vi "GeoData.vi"() -> ()   [LabVIEW 2017] (continued)
\t6079\tSan luis obispo\tCA\tSan Luis Obispo County\tH1\n93445\t6079\tOceano\tCA\tSan Luis Obispo County\tH1\n93421\t6079\tArroyo grande\tCA\tSan Luis Obispo County\tH1\n93426\t6079\tBradley\tCA\tSan Luis Obispo County\tH1\n93443\t6079\tMorro bay\tCA\tSan Luis Obispo County\tH1\n93435\t6079\tHarmony\tCA\tSan Luis Obispo County\tH1\n93453\t6079\tSanta margarita\tCA\tSan Luis Obispo County\tH1\n93409\t6079\tSan luis obispo\tCA\tSan Luis Obispo County\tH1\n93428\t6079\tCambria\tCA\tSan Luis Obispo County\tH1\n93452\t6079\tSan simeon\tCA\tSan Luis Obispo County\tH1\n93424\t6079\tAvila beach\tCA\tSan Luis Obispo County\tH1\n93446\t6079\tPaso robles\tCA\tSan Luis Obispo County\tH1\n93430\t6079\tCayucos\tCA\tSan Luis Obispo County\tH1\n93444\t6079\tNipomo\tCA\tSan Luis Obispo County\tH1\n93408\t6079\tSan luis obispo\tCA\tSan Luis Obispo County\tH1\n93407\t6079\tSan luis obispo\tCA\tSan Luis Obispo County\tH1\n93410\t6079\tSan luis obispo\tCA\tSan Luis Obispo County\tH1\n93423\t6079\tAtascadero\tCA\tSan Luis Obispo County\tH1\n93449\t6079\tPismo beach\tCA\tSan Luis Obispo County\tH1\n93465\t6079\tTempleton\tCA\tSan Luis Obispo County\tH1\n93461\t6079\tShandon\tCA\tSan Luis Obispo County\tH1\n93254\t6079\tNew cuyama\tCA\tSan Luis Obispo County\tH1\n93405\t6079\tSan luis obispo\tCA\tSan Luis Obispo County\tH1\n93402\t6079\tLos osos\tCA\tSan Luis Obispo County\tH1\n93442\t6079\tMorro bay\tCA\tSan Luis Obispo County\tH1\n93422\t6079\tAtascadero\tCA\tSan Luis Obispo County\tH1\n93432\t6079\tCreston\tCA\tSan Luis Obispo County\tH1\n93403\t6079\tSan luis obispo\tCA\tSan Luis Obispo County\tH1\n93412\t6079\tLos osos\tCA\tSan Luis Obispo County\tH1\n93433\t6079\tGrover beach\tCA\tSan Luis Obispo County\tH1\n93454\t6079\tSanta maria\tCA\tSan Luis Obispo County\tH1\n93458\t6079\tSanta maria\tCA\tSan Luis Obispo County\tH1\n93252\t6079\tMaricopa\tCA\tSan Luis Obispo County\tH1\n93451\t6079\tSan miguel\tCA\tSan Luis Obispo County\tH1\n93447\t6079\tPaso robles\tCA\tSan Luis Obispo County\tH1\n93448\t6079\tPismo beach\tCA\tSan Luis Obispo County\tH1\n93483\t6079\tGrover beach\tCA\tSan Luis Obispo County\tH1\n93401\t6079\tSan luis obispo\tCA\tSan Luis Obispo County\tH1\n93475\t6079\tOceano\tCA\tSan Luis Obispo County\tH1\n94404\t6081\tSan mateo\tCA\tSan Mateo County\tH1\n94128\t6081\tSan francisco\tCA\tSan Mateo County\tH1\n94011\t6081\tBurlingame\tCA\tSan Mateo County\tH1\n94017\t6081\tDaly city\tCA\tSan Mateo County\tH1\n94080\t6081\tSouth san francisco\tCA\tSan Mateo County\tH1\n94070\t6081\tSan carlos\tCA\tSan Mateo County\tH1\n94014\t6081\tDaly city\tCA\tSan Mateo County\tH1\n94025\t6081\tMenlo park\tCA\tSan Mateo County\tH1\n94030\t6081\tMillbrae\tCA\tSan Mateo County\tH1\n94044\t6081\tPacifica\tCA\tSan Mateo County\tH1\n94065\t6081\tRedwood city\tCA\tSan Mateo County\tH1\n94497\t6081\tSan mateo\tCA\tSan Mateo County\tH1\n94066\t6081\tSan bruno\tCA\tSan Mateo County\tH1\n94027\t6081\tAtherton\tCA\tSan Mateo County\tH1\n94021\t6081\tLoma mar\tCA\tSan Mateo County\tH1\n94401\t6081\tSan mateo\tCA\tSan Mateo County\tH1\n94002\t6081\tBelmont\tCA\tSan Mateo County\tH1\n94010\t6081\tBurlingame\tCA\tSan Mateo County\tH1\n94028\t6081\tPortola valley\tCA\tSan Mateo County\tH1\n94063\t6081\tRedwood city\tCA\tSan Mateo County\tH1\n94125\t6081\tSan francisco\tCA\tSan Mateo County\tH1\n94303\t6081\tPalo alto\tCA\tSan Mateo County\tH1\n94134\t6081\tSan francisco\tCA\tSan Mateo County\tH1\n94015\t6081\tDaly city\tCA\tSan Mateo County\tH1\n94018\t6081\tEl granada\tCA\tSan Mateo County\tH1\n94074\t6081\tSan gregorio\tCA\tSan Mateo County\tH1\n94026\t6081\tMenlo park\tCA\tSan Mateo County\tH1\n94112\t6081\tSan francisco\tCA\tSan Mateo County\tH1\n94403\t6081\tSan mateo\tCA\tSan Mateo County\tH1\n94019\t6081\tHalf moon bay\tCA\tSan Mateo County\tH1\n94038\t6081\tMoss beach\tCA\tSan Mateo County\tH1\n94402\t6081\tSan mateo\tCA\tSan Mateo County\tH1\n94005\t6081\tBrisbane\tCA\tSan Mateo County\tH1\n94064\t6081\tRedwood city\tCA\tSan Mateo County\tH1\n94020\t6081\tLa honda\tCA\tSan Mateo County\tH1\n94061\t6081\tRedwood city\tCA\tSan Mateo County\tH1\n94062\t6081\tRedwood city\tCA\tSan Mateo County\tH1\n94037\t6081\tMontara\tCA\tSan Mateo County\tH1\n94083\t6081\tSouth san francisco\tCA\tSan Mateo County\tH1\n94060\t6081\tPescadero\tCA\tSan Mateo County\tH1\n93105\t6083\tSanta barbara\tCA\tSanta Barbara County\tH1\n93116\t6083\tGoleta\tCA\tSanta Barbara County\tH1\n93437\t6083\tLompoc\tCA\tSanta Barbara County\tH1\n93102\t6083\tSanta barbara\tCA\tSanta Barbara County\tH1\n93120\t6083\tSanta barbara\tCA\tSanta Barbara County\tH1\n93440\t6083\tLos alamos\tCA\tSanta Barbara County\tH1\n93427\t6083\tBuellton\tCA\tSanta Barbara County\tH1\n93101\t6083\tSanta barbara\tCA\tSanta Barbara County\tH1\n93118\t6083\tGoleta\tCA\tSanta Barbara County\tH1\n93160\t6083\tSanta barbara\tCA\tSanta Barbara County\tH1\n93441\t6083\tLos olivos\tCA\tSanta Barbara County\tH1\n93436\t6083\tLompoc\tCA\tSanta Barbara County\tH1\n93109\t6083\tSanta barbara\tCA\tSanta Barbara County\tH1\n93111\t6083\tSanta barbara\tCA\tSanta Barbara County\tH1\n93106\t6083\tSanta barbara\tCA\tSanta Barbara County\tH1\n93254\t6083\tNew cuyama\tCA\tSanta Barbara County\tH1\n93429\t6083\tCasmalia\tCA\tSanta Barbara County\tH1\n93013\t6083\tCarpinteria\tCA\tSanta Barbara County\tH1\n93455\t6083\tSanta maria\tCA\tSanta Barbara County\tH1\n93190\t6083\tSanta barbara\tCA\tSanta Barbara County\tH1\n93110\t6083\tSanta barbara\tCA\tSanta Barbara County\tH1\n93108\t6083\tSanta barbara\tCA\tSanta Barbara County\tH1\n93457\t6083\tSanta maria\tCA\tSanta Barbara County\tH1\n93438\t6083\tLompoc\tCA\tSanta Barbara County\tH1\n93014\t6083\tCarpinteria\tCA\tSanta Barbara County\tH1\n93434\t6083\tGuadalupe\tCA\tSanta Barbara County\tH1\n93454\t6083\tSanta maria\tCA\tSanta Barbara County\tH1\n93463\t6083\tSolvang\tCA\tSanta Barbara County\tH1\n93458\t6083\tSanta maria\tCA\tSanta Barbara County\tH1\n93456\t6083\tSanta maria\tCA\tSanta Barbara County\tH1\n93252\t6083\tMaricopa\tCA\tSanta Barbara County\tH1\n93117\t6083\tGoleta\tCA\tSanta Barbara County\tH1\n93130\t6083\tSanta barbara\tCA\tSanta Barbara County\tH1\n93150\t6083\tSanta barbara\tCA\tSanta Barbara County\tH1\n93464\t6083\tSolvang\tCA\tSanta Barbara County\tH1\n93460\t6083\tSanta ynez\tCA\tSanta Barbara County\tH1\n93103\t6083\tSanta barbara\tCA\tSanta Barbara County\tH1\n93140\t6083\tSanta barbara\tCA\tSanta Barbara County\tH1\n93121\t6083\tSanta barbara\tCA\tSanta Barbara County\tH1\n93067\t6083\tSummerland\tCA\tSanta Barbara County\tH1\n93199\t6083\tGoleta\tCA\tSanta Barbara County\tH1\n94550\t6085\tLivermore\tCA\tSanta Clara County\tH1\n94040\t6085\tMountain view\tCA\tSanta Clara County\tH1\n95033\t6085\tLos gatos\tCA\tSanta Clara County\tH1\n95111\t6085\tSan jose\tCA\tSanta Clara County\tH1\n95113\t6085\tSan jose\tCA\tSanta Clara County\tH1\n95132\t6085\tSan jose\tCA\tSanta Clara County\tH1\n95122\t6085\tSan jose\tCA\tSanta Clara County\tH1\n95138\t6085\tSan jose\tCA\tSanta Clara County\tH1\n95150\t6085\tSan jose\tCA\tSanta Clara County\tH1\n95172\t6085\tSan jose\tCA\tSanta Clara County\tH1\n95071\t6085\tSaratoga\tCA\tSanta Clara County\tH1\n95164\t6085\tSan jose\tCA\tSanta Clara County\tH1\n95109\t6085\tSan jose\tCA\tSanta Clara County\tH1\n95141\t6085\tSan jose\tCA\tSanta Clara County\tH1\n94089\t6085\tSunnyvale\tCA\tSanta Clara County\tH1\n94301\t6085\tPalo alto\tCA\tSanta Clara County\tH1\n95030\t6085\tLos gatos\tCA\tSanta Clara County\tH1\n95119\t6085\tSan jose\tCA\tSanta Clara County\tH1\n95121\t6085\tSan jose\tCA\tSanta Clara County\tH1\n95156\t6085\tSan jose\tCA\tSanta Clara County\tH1\n95101\t6085\tSan jose\tCA\tSanta Clara County\tH1\n94306\t6085\tPalo alto\tCA\tSanta Clara County\tH1\n94024\t6085\tLos altos\tCA\tSanta Clara County\tH1\n95035\t6085\tMilpitas\tCA\tSanta Clara County\tH1\n95070\t6085\tSaratoga\tCA\tSanta Clara County\tH1\n95129\t6085\tSan jose\tCA\tSanta Clara County\tH1\n95130\t6085\tSan jose\tCA\tSanta Clara County\tH1\n95127\t6085\tSan jose\tCA\tSanta Clara County\tH1\n95123\t6085\tSan jose\tCA\tSanta Clara County\tH1\n95153\t6085\tSan jose\tCA\tSanta Clara County\tH1\n95002\t6085\tAlviso\tCA\tSanta Clara County\tH1\n95154\t6085\tSan jose\tCA\tSanta Clara County\tH1\n94085\t6085\tSunnyvale\tCA\tSanta Clara County\tH1\n94304\t6085\tPalo alto\tCA\tSanta Clara County\tH1\n94028\t6085\tPortola valley\tCA\tSanta Clara County\tH1\n95037\t6085\tMorgan hill\tCA\tSanta Clara County\tH1\n95050\t6085\tSanta clara\tCA\tSanta Clara County\tH1\n95076\t6085\tWatsonville\tCA\tSanta Clara County\tH1\n95120\t6085\tSan jose\tCA\tSanta Clara County\tH1\n95118\t6085\tSan jose\tCA\tSanta Clara County\tH1\n95131\t6085\tSan jose\tCA\tSanta Clara County\tH1\n95170\t6085\tSan jose\tCA\tSanta Clara County\tH1\n95134\t6085\tSan jose\tCA\tSanta Clara County\tH1\n95135\t6085\tSan jose\tCA\tSanta Clara County\tH1\n95021\t6085\tGilroy\tCA\tSanta Clara County\tH1\n95011\t6085\tCampbell\tCA\tSanta Clara County\tH1\n95158\t6085\tSan jose\tCA\tSanta Clara County\tH1\n95157\t6085\tSan jose\tCA\tSanta Clara County\tH1\n94035\t6085\tMountain view\tCA\tSanta Clara County\tH1\n95191\t6085\tSan jose\tCA\tSanta Clara County\tH1\n95013\t6085\tCoyote\tCA\tSanta Clara County\tH1\n94087\t6085\tSunnyvale\tCA\tSanta Clara County\tH1\n94303\t6085\tPalo alto\tCA\tSanta Clara County\tH1\n95051\t6085\tSanta clara\tCA\tSanta Clara County\tH1\n95032\t6085\tLos gatos\tCA\tSanta Clara County\tH1\n95056\t6085\tSanta clara\tCA\tSanta Clara County\tH1\n95110\t6085\tSan jose\tCA\tSanta Clara County\tH1\n95124\t6085\tSan jose\tCA\tSanta Clara County\tH1\n95125\t6085\tSan jose\tCA\tSanta Clara County\tH1\n95044\t6085\tRedwood estates\tCA\tSanta Clara County\tH1\n95151\t6085\tSan jose\tCA\tSanta Clara County\tH1\n95155\t6085\tSan jose\tCA\tSanta Clara County\tH1\n95015\t6085\tCupertino\tCA\tSanta Clara County\tH1\n95055\t6085\tSanta clara\tCA\tSanta Clara County\tH1\n95103\t6085\tSan jose\tCA\tSanta Clara County\tH1\n94086\t6085\tSunnyvale\tCA\tSanta Clara County\tH1\n95008\t6085\tCampbell\tCA\tSanta Clara County\tH1\n94043\t6085\tMountain view\tCA\tSanta Clara County\tH1\n95054\t6085\tSanta clara\tCA\tSanta Clara County\tH1\n95112\t6085\tSan jose\tCA\tSanta Clara County\tH1\n95117\t6085\tSan jose\tCA\tSanta Clara County\tH1\n95136\t6085\tSan jose\tCA\tSanta Clara County\tH1\n95026\t6085\tHoly city\tCA\tSanta Clara County\tH1\n95009\t6085\tCampbell\tCA\tSanta Clara County\tH1\n94088\t6085\tSunnyvale\tCA\tSanta Clara County\tH1\n95052\t6085\tSanta clara\tCA\tSanta Clara County\tH1\n94042\t6085\tMountain view\tCA\tSanta Clara County\tH1\n94039\t6085\tMountain view\tCA\tSanta Clara County\tH1\n95192\t6085\tSan jose\tCA\tSanta Clara County\tH1\n94023\t6085\tLos altos\tCA\tSanta Clara County\tH1\n95046\t6085\tSan martin\tCA\tSanta Clara County\tH1\n95023\t6085\tHollister\tCA\tSanta Clara County\tH1\n95116\t6085\tSan jose\tCA\tSanta Clara County\tH1\n95126\t6085\tSan jose\tCA\tSanta Clara County\tH1\n95159\t6085\tSan jose\tCA\tSanta Clara County\tH1\n95036\t6085\tMilpitas\tCA\tSanta Clara County\tH1\n94020\t6085\tLa honda\tCA\tSanta Clara County\tH1\n95161\t6085\tSan jose\tCA\tSanta Clara County\tH1\n95152\t6085\tSan jose\tCA\tSanta Clara County\tH1\n94302\t6085\tPalo alto\tCA\tSanta Clara County\tH1\n94305\t6085\tStanford\tCA\tSanta Clara County\tH1\n94022\t6085\tLos altos\tCA\tSanta Clara County\tH1\n94041\t6085\tMountain view\tCA\tSanta Clara County\tH1\n95020\t6085\tGilroy\tCA\tSanta Clara County\tH1\n95014\t6085\tCupertino\tCA\tSanta Clara County\tH1\n95038\t6085\tMorgan hill\tCA\tSanta Clara County\tH1\n95128\t6085\tSan jose\tCA\tSanta Clara County\tH1\n95133\t6085\tSan jose\tCA\tSanta Clara County\tH1\n95148\t6085\tSan jose\tCA\tSanta Clara County\tH1\n95140\t6085\tMount hamilton\tCA\tSanta Clara County\tH1\n95031\t6085\tLos gatos\tCA\tSanta Clara County\tH1\n95173\t6085\tSan jose\tCA\tSanta Clara County\tH1\n95139\t6085\tSan jose\tCA\tSanta Clara County\tH1\n95108\t6085\tSan jose\tCA\tSanta Clara County\tH1\n95160\t6085\tSan jose\tCA\tSanta Clara County\tH1\n95106\t6085\tSan jose\tCA\tSanta Clara County\tH1\n95033\t6087\tLos gatos\tCA\tSanta Cruz County\tH1\n95010\t6087\tCapitola\tCA\tSanta Cruz County\tH1\n95061\t6087\tSanta cruz\tCA\tSanta Cruz County\tH1\n95017\t6087\tDavenport\tCA\tSanta Cruz County\tH1\n95077\t6087\tWatsonville\tCA\tSanta Cruz County\tH1\n95006\t6087\tBoulder creek\tCA\tSanta Cruz County\tH1\n95062\t6087\tSanta cruz\tCA\tSanta Cruz County\tH1\n95076\t6087\tWatsonville\tCA\tSanta Cruz County\tH1\n95019\t6087\tFreedom\tCA\tSanta Cruz County\tH1\n95007\t6087\tBrookdale\tCA\tSanta Cruz County\tH1\n95073\t6087\tSoquel\tCA\tSanta Cruz County\tH1\n95041\t6087\tMount hermon\tCA\tSanta Cruz County\tH1\n95060\t6087\tSanta cruz\tCA\tSanta Cruz County\tH1\n95065\t6087\tSanta cruz\tCA\tSanta Cruz County\tH1\n95003\t6087\tAptos\tCA\tSanta Cruz County\tH1\n95005\t6087\tBen lomond\tCA\tSanta Cruz County\tH1\n95018\t6087\tFelton\tCA\tSanta Cruz County\tH1\n95001\t6087\tAptos\tCA\tSanta Cruz County\tH1\n95067\t6087\tScotts valley\tCA\tSanta Cruz County\tH1\n95066\t6087\tScotts valley\tCA\tSanta Cruz County\tH1\n95063\t6087\tSanta cruz\tCA\tSanta Cruz County\tH1\n94060\t6087\tPescadero\tCA\tSanta Cruz County\tH1\n95064\t6087\tSanta cruz\tCA\tSanta Cruz County\tH1\n96001\t6089\tRedding\tCA\tShasta County\tH1\n96022\t6089\tCottonwood\tCA\tShasta County\tH1\n96062\t6089\tMillville\tCA\tShasta County\tH1\n96076\t6089\tPlatina\tCA\tShasta County\tH1\n96099\t6089\tRedding\tCA\tShasta County\tH1\n96051\t6089\tLakehead\tCA\tShasta County\tH1\n96019\t6089\tShasta lake\tCA\tShasta County\tH1\n96096\t6089\tWhitmore\tCA\tShasta County\tH1\n96047\t6089\tIgo\tCA\tShasta County\tH1\n96040\t6089\tHat creek\tCA\tShasta County\tH1\n96087\t6089\tShasta\tCA\tShasta County\tH1\n96095\t6089\tWhiskeytown\tCA\tShasta County\tH1\n96089\t6089\tShasta lake\tCA\tShasta County\tH1\n96002\t6089\tRedding\tCA\tShasta County\tH1\n96073\t6089\tPalo cedro\tCA\tShasta County\tH1\n96017\t6089\tCastella\tCA\tShasta County\tH1\n96049\t6089\tRedding\tCA\tShasta County\tH1\n96069\t6089\tOak run\tCA\tShasta County\tH1\n96011\t6089\tBig bend\tCA\tShasta County\tH1\n96056\t6089\tMcarthur\tCA\tShasta County\tH1\n96059\t6089\tManton\tCA\tShasta County\tH1\n96071\t6089\tOld station\tCA\tShasta County\tH1\n96007\t6089\tAnderson\tCA\tShasta County\tH1\n96028\t6089\tFall river mills\tCA\tShasta County\tH1\n96088\t6089\tShingletown\tCA\tShasta County\tH1\n96065\t6089\tMontgomery creek\tCA\tShasta County\tH1\n96033\t6089\tFrench gulch\tCA\tShasta County\tH1\n96016\t6089\tCassel\tCA\tShasta County\tH1\n96084\t6089\tRound mountain\tCA\tShasta County\tH1\n96025\t6089\tDunsmuir\tCA\tShasta County\tH1\n96008\t6089\tBella vista\tCA\tShasta County\tH1\n96003\t6089\tRedding\tCA\tShasta County\tH1\n96013\t6089\tBurney\tCA\tShasta County\tH1\n96118\t6091\tLoyalton\tCA\tSierra County\tH1\n95922\t6091\tCamptonville\tCA\tSierra County\tH1\n95910\t6091\tAlleghany\tCA\tSierra County\tH1\n96125\t6091\tSierra city\tCA\tSierra County\tH1\n95936\t6091\tDownieville\tCA\tSierra County\tH1\n95960\t6091\tNorth san juan\tCA\tSierra County\tH1\n96124\t6091\tCalpine\tCA\tSierra County\tH1\n95944\t6091\tGoodyears bar\tCA\tSierra County\tH1\n96126\t6091\tSierraville\tCA\tSierra County\tH1\n96134\t6093\tTulelake\tCA\tSiskiyou County\tH1\n96031\t6093\tForks of salmon\tCA\tSiskiyou County\tH1\n96085\t6093\tScott bar\tCA\tSiskiyou County\tH1\n96067\t6093\tMount shasta\tCA\tSiskiyou County\tH1\n96014\t6093\tCallahan\tCA\tSiskiyou County\tH1\n96038\t6093\tGrenada\tCA\tSiskiyou County\tH1\n96097\t6093\tYreka\tCA\tSiskiyou County\tH1\n96032\t6093\tFort jones\tCA\tSiskiyou County\tH1\n96058\t6093\tMacdoel\tCA\tSiskiyou County\tH1\n96086\t6093\tSeiad valley\tCA\tSiskiyou County\tH1\n96094\t6093\tWeed\tCA\tSiskiyou County\tH1\n96044\t6093\tHornbrook\tCA\tSiskiyou County\tH1\n96039\t6093\tHappy camp\tCA\tSiskiyou County\tH1\n96037\t6093\tGreenview\tCA\tSiskiyou County\tH1\n96025\t6093\tDunsmuir\tCA\tSiskiyou County\tH1\n96027\t6093\tEtna\tCA\tSiskiyou County\tH1\n96050\t6093\tKlamath river\tCA\tSiskiyou County\tH1\n96064\t6093\tMontague\tCA\tSiskiyou County\tH1\n96034\t6093\tGazelle\tCA\tSiskiyou County\tH1\n95568\t6093\tSomes bar\tCA\tSiskiyou County\tH1\n96023\t6093\tDorris\tCA\tSiskiyou County\tH1\n96057\t6093\tMccloud\tCA\tSiskiyou County\tH1\n94590\t6095\tVallejo\tCA\tSolano County\tH1\n95616\t6095\tDavis\tCA\tSolano County\tH1\n95690\t6095\tWalnut grove\tCA\tSolano County\tH1\n94533\t6095\tFairfield\tCA\tSolano County\tH1\n95688\t6095\tVacaville\tCA\tSolano County\tH1\n94558\t6095\tNapa\tCA\tSolano County\tH1\n94512\t6095\tBirds landing\tCA\tSolano County\tH1\n94503\t6095\tAmerican canyon\tCA\tSolano County\tH1\n95618\t6095\tDavis\tCA\tSolano County\tH1\n95620\t6095\tDixon\tCA\tSolano County\tH1\n95696\t6095\tVacaville\tCA\tSolano County\tH1\n94592\t6095\tVallejo\tCA\tSolano County\tH1\n94589\t6095\tVallejo\tCA\tSolano County\tH1\n94591\t6095\tVallejo\tCA\tSolano County\tH1\n95625\t6095\tElmira\tCA\tSolano County\tH1\n94510\t6095\tBenicia\tCA\tSolano County\tH1\n94571\t6095\tRio vista\tCA\tSolano County\tH1\n95687\t6095\tVacaville\tCA\tSolano County\tH1\n94535\t6095\tTravis afb\tCA\tSolano County\tH1\n94585\t6095\tSuisun city\tCA\tSolano County\tH1\n95694\t6095\tWinters\tCA\tSolano County\tH1\n94534\t6095\tFairfield\tCA\tSolano County\tH1\n95448\t6097\tHealdsburg\tCA\tSonoma County\tH1\n94574\t6097\tSaint helena\tCA\tSonoma County\tH1\n95452\t6097\tKenwood\tCA\tSonoma County\tH1\n95416\t6097\tBoyes hot springs\tCA\tSonoma County\tH1\n94953\t6097\tPetaluma\tCA\tSonoma County\tH1\n95425\t6097\tCloverdale\tCA\tSonoma County\tH1\n94515\t6097\tCalistoga\tCA\tSonoma County\tH1\n95405\t6097\tSanta rosa\tCA\tSonoma County\tH1\n95441\t6097\tGeyserville\tCA\tSonoma County\tH1\n95419\t6097\tCamp meeker\tCA\tSonoma County\tH1\n94975\t6097\tPetaluma\tCA\tSonoma County\tH1\n95430\t6097\tDuncans mills\tCA\tSonoma County\tH1\n95421\t6097\tCazadero\tCA\tSonoma County\tH1\n94558\t6097\tNapa\tCA\tSonoma County\tH1\n94931\t6097\tCotati\tCA\tSonoma County\tH1\n95412\t6097\tAnnapolis\tCA\tSonoma County\tH1\n94955\t6097\tPetaluma\tCA\tSonoma County\tH1\n95444\t6097\tGraton\tCA\tSonoma County\tH1\n95487\t6097\tVineburg\tCA\tSonoma County\tH1\n95486\t6097\tVilla grande\tCA\tSonoma County\tH1\n94928\t6097\tRohnert park\tCA\tSonoma County\tH1\n95404\t6097\tSanta rosa\tCA\tSonoma County\tH1\n95402\t6097\tSanta rosa\tCA\tSonoma County\tH1\n95465\t6097\tOccidental\tCA\tSonoma County\tH1\n95497\t6097\tThe sea ranch\tCA\tSonoma County\tH1\n95476\t6097\tSonoma\tCA\tSonoma County\tH1\n95442\t6097\tGlen ellen\tCA\tSonoma County\tH1\n95436\t6097\tForestville\tCA\tSonoma County\tH1\n95461\t6097\tMiddletown\tCA\tSonoma County\tH1\n94952\t6097\tPetaluma\tCA\tSonoma County\tH1\n95403\t6097\tSanta rosa\tCA\tSonoma County\tH1\n94954\t6097\tPetaluma\tCA\tSonoma County\tH1\n95433\t6097\tEl verano\tCA\tSonoma County\tH1\n94923\t6097\tBodega bay\tCA\tSonoma County\tH1\n95450\t6097\tJenner\tCA\tSonoma County\tH1\n95471\t6097\tRio nido\tCA\tSonoma County\tH1\n95473\t6097\tSebastopol\tCA\tSonoma County\tH1\n94972\t6097\tValley ford\tCA\tSonoma County\tH1\n95407\t6097\tSanta rosa\tCA\tSonoma County\tH1\n94945\t6097\tNovato\tCA\tSonoma County\tH1\n95462\t6097\tMonte rio\tCA\tSonoma County\tH1\n94922\t6097\tBodega\tCA\tSonoma County\tH1\n95431\t6097\tEldridge\tCA\tSonoma County\tH1\n95472\t6097\tSebastopol\tCA\tSonoma County\tH1\n95445\t6097\tGualala\tCA\tSonoma County\tH1\n95401\t6097\tSanta rosa\tCA\tSonoma County\tH1\n94951\t6097\tPenngrove\tCA\tSonoma County\tH1\n95406\t6097\tSanta rosa\tCA\tSonoma County\tH1\n94927\t6097\tRohnert park\tCA\tSonoma County\tH1\n95480\t6097\tStewarts point\tCA\tSonoma County\tH1\n94999\t6097\tPetaluma\tCA\tSonoma County\tH1\n95409\t6097\tSanta rosa\tCA\tSonoma County\tH1\n95492\t6097\tWindsor\tCA\tSonoma County\tH1\n95446\t6097\tGuerneville\tCA\tSonoma County\tH1\n95439\t6097\tFulton\tCA\tSonoma County\tH1\n94550\t6099\tLivermore\tCA\tStanislaus County\tH1\n95351\t6099\tModesto\tCA\tStanislaus County\tH1\n95352\t6099\tModesto\tCA\tStanislaus County\tH1\n95354\t6099\tModesto\tCA\tStanislaus County\tH1\n95353\t6099\tModesto\tCA\tStanislaus County\tH1\n95313\t6099\tCrows landing\tCA\tStanislaus County\tH1\n95382\t6099\tTurlock\tCA\tStanislaus County\tH1\n95358\t6099\tModesto\tCA\tStanislaus County\tH1\n95360\t6099\tNewman\tCA\tStanislaus County\tH1\n95385\t6099\tVernalis\tCA\tStanislaus County\tH1\n95356\t6099\tModesto\tCA\tStanislaus County\tH1\n95328\t6099\tKeyes\tCA\tStanislaus County\tH1\n95323\t6099\tHickman\tCA\tStanislaus County\tH1\n95319\t6099\tEmpire\tCA\tStanislaus County\tH1\n95387\t6099\tWestley\tCA\tStanislaus County\tH1\n95326\t6099\tHughson\tCA\tStanislaus County\tH1\n95350\t6099\tModesto\tCA\tStanislaus County\tH1\n95316\t6099\tDenair\tCA\tStanislaus County\tH1\n95386\t6099\tWaterford\tCA\tStanislaus County\tH1\n95322\t6099\tGustine\tCA\tStanislaus County\tH1\n95357\t6099\tModesto\tCA\tStanislaus County\tH1\n95324\t6099\tHilmar\tCA\tStanislaus County\tH1\n95363\t6099\tPatterson\tCA\tStanislaus County\tH1\n95380\t6099\tTurlock\tCA\tStanislaus County\tH1\n95307\t6099\tCeres\tCA\tStanislaus County\tH1\n95329\t6099\tLa grange\tCA\tStanislaus County\tH1\n95367\t6099\tRiverbank\tCA\tStanislaus County\tH1\n95397\t6099\tModesto\tCA\tStanislaus County\tH1\n95355\t6099\tModesto\tCA\tStanislaus County\tH1\n95361\t6099\tOakdale\tCA\tStanislaus County\tH1\n95368\t6099\tSalida\tCA\tStanislaus County\tH1\n95381\t6099\tTurlock\tCA\tStanislaus County\tH1\n95230\t6099\tFarmington\tCA\tStanislaus County\tH1\n95645\t6101\tKnights landing\tCA\tSutter County\tH1\n95948\t6101\tGridley\tCA\tSutter County\tH1\n95991\t6101\tYuba city\tCA\tSutter County\tH1\n95993\t6101\tYuba city\tCA\tSutter County\tH1\n95626\t6101\tElverta\tCA\tSutter County\tH1\n95674\t6101\tRio oso\tCA\tSutter County\tH1\n95982\t6101\tSutter\tCA\tSutter County\tH1\n95659\t6101\tNicolaus\tCA\tSutter County\tH1\n95836\t6101\tSacramento\tCA\tSutter County\tH1\n95676\t6101\tRobbins\tCA\tSutter County\tH1\n95837\t6101\tSacramento\tCA\tSutter County\tH1\n95692\t6101\tWheatland\tCA\tSutter County\tH1\n95957\t6101\tMeridian\tCA\tSutter County\tH1\n95953\t6101\tLive oak\tCA\tSutter County\tH1\n95992\t6101\tYuba city\tCA\tSutter County\tH1\n95668\t6101\tPleasant grove\tCA\tSutter County\tH1\n96022\t6103\tCottonwood\tCA\tTehama County\tH1\n96078\t6103\tProberta\tCA\tTehama County\tH1\n96021\t6103\tCorning\tCA\tTehama County\tH1\n96076\t6103\tPlatina\tCA\tTehama County\tH1\n96063\t6103\tMineral\tCA\tTehama County\tH1\n95963\t6103\tOrland\tCA\tTehama County\tH1\n95973\t6103\tChico\tCA\tTehama County\tH1\n96080\t6103\tRed bluff\tCA\tTehama County\tH1\n96059\t6103\tManton\tCA\tTehama County\tH1\n96090\t6103\tTehama\tCA\tTehama County\tH1\n96061\t6103\tMill creek\tCA\tTehama County\tH1\n96092\t6103\tVina\tCA\tTehama County\tH1\n96007\t6103\tAnderson\tCA\tTehama County\tH1\n96055\t6103\tLos molinos\tCA\tTehama County\tH1\n96035\t6103\tGerber\tCA\tTehama County\tH1\n96074\t6103\tPaskenta\tCA\tTehama County\tH1\n96029\t6103\tFlournoy\tCA\tTehama County\tH1\n96075\t6103\tPaynes creek\tCA\tTehama County\tH1\n95595\t6105\tZenia\tCA\tTrinity County\tH1\n96076\t6105\tPlatina\tCA\tTrinity County\tH1\n96046\t6105\tHyampom\tCA\tTrinity County\tH1\n95526\t6105\tBridgeville\tCA\tTrinity County\tH1\n96052\t6105\tLewiston\tCA\tTrinity County\tH1\n96091\t6105\tTrinity center\tCA\tTrinity County\tH1\n95527\t6105\tBurnt ranch\tCA\tTrinity County\tH1\n96093\t6105\tWeaverville\tCA\tTrinity County\tH1\n96024\t6105\tDouglas city\tCA\tTrinity County\tH1\n96041\t6105\tHayfork\tCA\tTrinity County\tH1\n95552\t6105\tMad river\tCA\tTrinity County\tH1\n96048\t6105\tJunction city\tCA\tTrinity County\tH1\n96010\t6105\tBig bar\tCA\tTrinity County\tH1\n93247\t6107\tLindsay\tCA\tTulare County\tH1\n93223\t6107\tFarmersville\tCA\tTulare County\tH1\n93286\t6107\tWoodlake\tCA\tTulare County\tH1\n93647\t6107\tOrosi\tCA\tTulare County\tH1\n93675\t6107\tSquaw valley\tCA\tTulare County\tH1\n93673\t6107\tTraver\tCA\tTulare County\tH1\n93244\t6107\tLemon cove\tCA\tTulare County\tH1\n93666\t6107\tSultana\tCA\tTulare County\tH1\n93215\t6107\tDelano\tCA\tTulare County\tH1\n93221\t6107\tExeter\tCA\tTulare County\tH1\n93258\t6107\tPorterville\tCA\tTulare County\tH1\n93291\t6107\tVisalia\tCA\tTulare County\tH1\n93256\t6107\tPixley\tCA\tTulare County\tH1\n93641\t6107\tMiramonte\tCA\tTulare County\tH1\n93278\t6107\tVisalia\tCA\tTulare County\tH1\n93275\t6107\tTulare\tCA\tTulare County\tH1\n93603\t6107\tBadger\tCA\tTulare County\tH1\n93290\t6107\tVisalia\tCA\tTulare County\tH1\n93654\t6107\tReedley\tCA\tTulare County\tH1\n93633\t6107\tKings canyon national pk\tCA\tTulare County\tH1\n93292\t6107\tVisalia\tCA\tTulare County\tH1\n93271\t6107\tThree rivers\tCA\tTulare County\tH1\n93274\t6107\tTulare\tCA\tTulare County\tH1\n93279\t6107\tVisalia\tCA\tTulare County\tH1\n93670\t6107\tYettem\tCA\tTulare County\tH1\n93615\t6107\tCutler\tCA\tTulare County\tH1\n93260\t6107\tPosey\tCA\tTulare County\tH1\n93218\t6107\tDucor\tCA\tTulare County\tH1\n93237\t6107\tKaweah\tCA\tTulare County\tH1\n93219\t6107\tEarlimart\tCA\tTulare County\tH1\n93230\t6107\tHanford\tCA\tTulare County\tH1\n93272\t6107\tTipton\tCA\tTulare County\tH1\n93618\t6107\tDinuba\tCA\tTulare County\tH1\n93646\t6107\tOrange cove\tCA\tTulare County\tH1\n93631\t6107\tKingsburg\tCA\tTulare County\tH1\n93208\t6107\tCamp nelson\tCA\tTulare County\tH1\n93261\t6107\tRichgrove\tCA\tTulare County\tH1\n93227\t6107\tGoshen\tCA\tTulare County\tH1\n93212\t6107\tCorcoran\tCA\tTulare County\tH1\n93235\t6107\tIvanhoe\tCA\tTulare County\tH1\n93262\t6107\tSequoia national park\tCA\tTulare County\tH1\n93201\t6107\tAlpaugh\tCA\tTulare County\tH1\n93257\t6107\tPorterville\tCA\tTulare County\tH1\n93277\t6107\tVisalia\tCA\tTulare County\tH1\n93267\t6107\tStrathmore\tCA\tTulare County\tH1\n93265\t6107\tSpringville\tCA\tTulare County\tH1\n93270\t6107\tTerra bella\tCA\tTulare County\tH1\n93207\t6107\tCalifornia hot springs\tCA\tTulare County\tH1\n95311\t6109\tCoulterville\tCA\tTuolumne County\tH1\n95373\t6109\tStandard\tCA\tTuolumne County\tH1\n95364\t6109\tPinecrest\tCA\tTuolumne County\tH1\n95305\t6109\tBig oak flat\tCA\tTuolumne County\tH1\n95321\t6109\tGroveland\tCA\tTuolumne County\tH1\n95310\t6109\tColumbia\tCA\tTuolumne County\tH1\n95383\t6109\tTwain harte\tCA\tTuolumne County\tH1\n95335\t6109\tLong barn\tCA\tTuolumne County\tH1\n95379\t6109\tTuolumne\tCA\tTuolumne County\tH1\n95327\t6109\tJamestown\tCA\tTuolumne County\tH1\n95370\t6109\tSonora\tCA\tTuolumne County\tH1\n95372\t6109\tSoulsbyville\tCA\tTuolumne County\tH1\n95347\t6109\tMoccasin\tCA\tTuolumne County\tH1\n95329\t6109\tLa grange\tCA\tTuolumne County\tH1\n95375\t6109\tStrawberry\tCA\tTuolumne County\tH1\n95309\t6109\tChinese camp\tCA\tTuolumne County\tH1\n95346\t6109\tMi wuk village\tCA\tTuolumne County\tH1\n91304\t6111\tCanoga park\tCA\tVentura County\tH1\n91307\t6111\tWest hills\tCA\tVentura County\tH1\n93015\t6111\tFillmore\tCA\tVentura County\tH1\n93023\t6111\tOjai\tCA\tVentura County\tH1\n93060\t6111\tSanta paula\tCA\tVentura County\tH1\n93034\t6111\tOxnard\tCA\tVentura County\tH1\n93024\t6111\tOjai\tCA\tVentura County\tH1\n91359\t6111\tWestlake village\tCA\tVentura County\tH1\n90265\t6111\tMalibu\tCA\tVentura County\tH1\n93004\t6111\tVentura\tCA\tVentura County\tH1\n93006\t6111\tVentura\tCA\tVentura County\tH1\n93012\t6111\tCamarillo\tCA\tVentura County\tH1\n93041\t6111\tPort hueneme\tCA\tVentura County\tH1\n93065\t6111\tSimi valley\tCA\tVentura County\tH1\n93043\t6111\tPort hueneme cbc base\tCA\tVentura County\tH1\n93064\t6111\tBrandeis\tCA\tVentura County\tH1\n93009\t6111\tVentura\tCA\tVentura County\tH1\n91320\t6111\tNewbury park\tCA\tVentura County\tH1\n93021\t6111\tMoorpark\tCA\tVentura County\tH1\n91361\t6111\tWestlake village\tCA\tVentura County\tH1\n91377\t6111\tOak park\tCA\tVentura County\tH1\n93031\t6111\tOxnard\tCA\tVentura County\tH1\n93040\t6111\tPiru\tCA\tVentura County\tH1\n93032\t6111\tOxnard\tCA\tVentura County\tH1\n93066\t6111\tSomis\tCA\tVentura County\tH1\n91360\t6111\tThousand oaks\tCA\tVentura County\tH1\n93010\t6111\tCamarillo\tCA\tVentura County\tH1\n93013\t6111\tCarpinteria\tCA\tVentura County\tH1\n93033\t6111\tOxnard\tCA\tVentura County\tH1\n93036\t6111\tOxnard\tCA\tVentura County\tH1\n93044\t6111\tPort hueneme\tCA\tVentura County\tH1\n93062\t6111\tSimi valley\tCA\tVentura County\tH1\n91358\t6111\tThousand oaks\tCA\tVentura County\tH1\n93042\t6111\tPoint mugu nawc\tCA\tVentura County\tH1\n93007\t6111\tVentura\tCA\tVentura County\tH1\n93001\t6111\tVentura\tCA\tVentura County\tH1\n93063\t6111\tSimi valley\tCA\tVentura County\tH1\n93252\t6111\tMaricopa\tCA\tVentura County\tH1\n91362\t6111\tThousand oaks\tCA\tVentura County\tH1\n91319\t6111\tNewbury park\tCA\tVentura County\tH1\n93094\t6111\tSimi valley\tCA\tVentura County\tH1\n93020\t6111\tMoorpark\tCA\tVentura County\tH1\n93016\t6111\tFillmore\tCA\tVentura County\tH1\n93030\t6111\tOxnard\tCA\tVentura County\tH1\n93011\t6111\tCamarillo\tCA\tVentura County\tH1\n93005\t6111\tVentura\tCA\tVentura County\tH1\n93061\t6111\tSanta paula\tCA\tVentura County\tH1\n91311\t6111\tChatsworth\tCA\tVentura County\tH1\n93003\t6111\tVentura\tCA\tVentura County\tH1\n93002\t6111\tVentura\tCA\tVentura County\tH1\n93022\t6111\tOak view\tCA\tVentura County\tH1\n93035\t6111\tOxnard\tCA\tVentura County\tH1\n93225\t6111\tFrazier park\tCA\tVentura County\tH1\n93099\t6111\tSimi valley\tCA\tVentura County\tH1\n95616\t6113\tDavis\tCA\tYolo County\tH1\n95645\t6113\tKnights landing\tCA\tYolo County\tH1\n95697\t6113\tYolo\tCA\tYolo County\tH1\n95691\t6113\tWest sacramento\tCA\tYolo County\tH1\n95627\t6113\tEsparto\tCA\tYolo County\tH1\n95637\t6113\tGuinda\tCA\tYolo County\tH1\n95618\t6113\tDavis\tCA\tYolo County\tH1\n95620\t6113\tDixon\tCA\tYolo County\tH1\n95799\t6113\tWest sacramento\tCA\tYolo County\tH1\n95695\t6113\tWoodland\tCA\tYolo County\tH1\n95612\t6113\tClarksburg\tCA\tYolo County\tH1\n95607\t6113\tCapay\tCA\tYolo County\tH1\n95606\t6113\tBrooks\tCA\tYolo County\tH1\n95937\t6113\tDunnigan\tCA\tYolo County\tH1\n95653\t6113\tMadison\tCA\tYolo County\tH1\n95617\t6113\tDavis\tCA\tYolo County\tH1\n95694\t6113\tWinters\tCA\tYolo County\tH1\n95912\t6113\tArbuckle\tCA\tYolo County\tH1\n95798\t6113\tWest sacramento\tCA\tYolo County\tH1\n95615\t6113\tCourtland\tCA\tYolo County\tH1\n95679\t6113\tRumsey\tCA\tYolo County\tH1\n95698\t6113\tZamora\tCA\tYolo County\tH1\n95605\t6113\tWest sacramento\tCA\tYolo County\tH1\n95776\t6113\tWoodland\tCA\tYolo County\tH1\n95977\t6115\tSmartsville\tCA\tYuba County\tH1\n95935\t6115\tDobbins\tCA\tYuba County\tH1\n95901\t6115\tMarysville\tCA\tYuba County\tH1\n95914\t6115\tBangor\tCA\tYuba County\tH1\n95925\t6115\tChallenge\tCA\tYuba County\tH1\n95962\t6115\tOregon house\tCA\tYuba County\tH1\n95972\t6115\tRackerby\tCA\tYuba County\tH1\n95903\t6115\tBeale afb\tCA\tYuba County\tH1\n95922\t6115\tCamptonville\tCA\tYuba County\tH1\n95981\t6115\tStrawberry valley\tCA\tYuba County\tH1\n95961\t6115\tOlivehurst\tCA\tYuba County\tH1\n95692\t6115\tWheatland\tCA\tYuba County\tH1\n95941\t6115\tForbestown\tCA\tYuba County\tH1\n95960\t6115\tNorth san juan\tCA\tYuba County\tH1\n95919\t6115\tBrownsville\tCA\tYuba County\tH1\n95966\t6115\tOroville\tCA\tYuba County\tH1\n95918\t6115\tBrowns valley\tCA\tYuba County\tH1\n80229\t8001\tDenver\tCO\tAdams County\tH1\n80701\t8001\tFort morgan\tCO\tAdams County\tH1\n80642\t8001\tHudson\tCO\tAdams County\tH1\n80654\t8001\tWiggins\tCO\tAdams County\tH1\n80247\t8001\tDenver\tCO\tAdams County\tH1\n80266\t8001\tDenver\tCO\tAdams County\tH1\n80221\t8001\tDenver\tCO\tAdams County\tH1\n80640\t8001\tHenderson\tCO\tAdams County\tH1\n80002\t8001\tArvada\tCO\tAdams County\tH1\n80105\t8001\tDeer trail\tCO\tAdams County\tH1\n80042\t8001\tAurora\tCO\tAdams County\tH1\n80102\t8001\tBennett\tCO\tAdams County\tH1\n80045\t8001\tAurora\tCO\tAdams County\tH1\n80239\t8001\tDenver\tCO\tAdams County\tH1\n80220\t8001\tDenver\tCO\tAdams County\tH1\n80602\t8001\tBrighton\tCO\tAdams County\tH1\n80036\t8001\tWestminster\tCO\tAdams County\tH1\n80003\t8001\tArvada\tCO\tAdams County\tH1\n80011\t8001\tAurora\tCO\tAdams County\tH1\n80010\t8001\tAurora\tCO\tAdams County\tH1\n80020\t8001\tBroomfield\tCO\tAdams County\tH1\n80023\t8001\tBroomfield\tCO\tAdams County\tH1\n80022\t8001\tCommerce city\tCO\tAdams County\tH1\n80136\t8001\tStrasburg\tCO\tAdams County\tH1\n80212\t8001\tDenver\tCO\tAdams County\tH1\n80234\t8001\tDenver\tCO\tAdams County\tH1\n80037\t8001\tCommerce city\tCO\tAdams County\tH1\n80035\t8001\tWestminster\tCO\tAdams County\tH1\n80031\t8001\tWestminster\tCO\tAdams County\tH1\n80233\t8001\tDenver\tCO\tAdams County\tH1\n80601\t8001\tBrighton\tCO\tAdams County\tH1\n80643\t8001\tKeenesburg\tCO\tAdams County\tH1\n80238\t8001\tDenver\tCO\tAdams County\tH1\n80241\t8001\tThornton\tCO\tAdams County\tH1\n80614\t8001\tEastlake\tCO\tAdams County\tH1\n80019\t8001\tAurora\tCO\tAdams County\tH1\n80024\t8001\tDupont\tCO\tAdams County\tH1\n80030\t8001\tWestminster\tCO\tAdams County\tH1\n80040\t8001\tAurora\tCO\tAdams County\tH1\n80137\t8001\tWatkins\tCO\tAdams County\tH1\n80249\t8001\tDenver\tCO\tAdams County\tH1\n80103\t8001\tByers\tCO\tAdams County\tH1\n80216\t8001\tDenver\tCO\tAdams County\tH1\n80603\t8001\tBrighton\tCO\tAdams County\tH1\n80260\t8001\tDenver\tCO\tAdams County\tH1\n81101\t8003\tAlamosa\tCO\tAlamosa County\tH1\n81102\t8003\tAlamosa\tCO\tAlamosa County\tH1\n81125\t8003\tCenter\tCO\tAlamosa County\tH1\n81136\t8003\tHooper\tCO\tAlamosa County\tH1\n81144\t8003\tMonte vista\tCO\tAlamosa County\tH1\n81146\t8003\tMosca\tCO\tAlamosa County\tH1\n80013\t8005\tAurora\tCO\tArapahoe County\tH1\n80017\t8005\tAurora\tCO\tArapahoe County\tH1\n80110\t8005\tEnglewood\tCO\tArapahoe County\tH1\n80113\t8005\tEnglewood\tCO\tArapahoe County\tH1\n80224\t8005\tDenver\tCO\tArapahoe County\tH1\n80247\t8005\tDenver\tCO\tArapahoe County\tH1\n80044\t8005\tAurora\tCO\tArapahoe County\tH1\n80161\t8005\tLittleton\tCO\tArapahoe County\tH1\n80155\t8005\tEnglewood\tCO\tArapahoe County\tH1\n80251\t8005\tDenver\tCO\tArapahoe County\tH1\n80112\t8005\tEnglewood\tCO\tArapahoe County\tH1\n80246\t8005\tDenver\tCO\tArapahoe County\tH1\n80046\t8005\tAurora\tCO\tArapahoe County\tH1\n80014\t8005\tAurora\tCO\tArapahoe County\tH1\n80015\t8005\tAurora\tCO\tArapahoe County\tH1\n80105\t8005\tDeer trail\tCO\tArapahoe County\tH1\n80102\t8005\tBennett\tCO\tArapahoe County\tH1\n80045\t8005\tAurora\tCO\tArapahoe County\tH1\n80210\t8005\tDenver\tCO\tArapahoe County\tH1\n80236\t8005\tDenver\tCO\tArapahoe County\tH1\n80012\t8005\tAurora\tCO\tArapahoe County\tH1\n80120\t8005\tLittleton\tCO\tArapahoe County\tH1\n80123\t8005\tLittleton\tCO\tArapahoe County\tH1\n80111\t8005\tEnglewood\tCO\tArapahoe County\tH1\n80129\t8005\tLittleton\tCO\tArapahoe County\tH1\n80220\t8005\tDenver\tCO\tArapahoe County\tH1\n80231\t8005\tDenver\tCO\tArapahoe County\tH1\n80011\t8005\tAurora\tCO\tArapahoe County\tH1\n80010\t8005\tAurora\tCO\tArapahoe County\tH1\n80121\t8005\tLittleton\tCO\tArapahoe County\tH1\n80138\t8005\tParker\tCO\tArapahoe County\tH1\n80047\t8005\tAurora\tCO\tArapahoe County\tH1\n80136\t8005\tStrasburg\tCO\tArapahoe County\tH1\n80222\t8005\tDenver\tCO\tArapahoe County\tH1\n80018\t8005\tAurora\tCO\tArapahoe County\tH1\n80016\t8005\tAurora\tCO\tArapahoe County\tH1\n80041\t8005\tAurora\tCO\tArapahoe County\tH1\n80230\t8005\tDenver\tCO\tArapahoe County\tH1\n80019\t8005\tAurora\tCO\tArapahoe County\tH1\n80151\t8005\tEnglewood\tCO\tArapahoe County\tH1\n80128\t8005\tLittleton\tCO\tArapahoe County\tH1\n80137\t8005\tWatkins\tCO\tArapahoe County\tH1\n80166\t8005\tLittleton\tCO\tArapahoe County\tH1\n80122\t8005\tLittleton\tCO\tArapahoe County\tH1\n80103\t8005\tByers\tCO\tArapahoe County\tH1\n80237\t8005\tDenver\tCO\tArapahoe County\tH1\n80160\t8005\tLittleton\tCO\tArapahoe County\tH1\n80150\t8005\tEnglewood\tCO\tArapahoe County\tH1\n80165\t8005\tLittleton\tCO\tArapahoe County\tH1\n81137\t8007\tIgnacio\tCO\tArchuleta County\tH1\n81157\t8007\tPagosa springs\tCO\tArchuleta County\tH1\n81128\t8007\tChromo\tCO\tArchuleta County\tH1\n81122\t8007\tBayfield\tCO\tArchuleta County\tH1\n81121\t8007\tArboles\tCO\tArchuleta County\tH1\n81147\t8007\tPagosa springs\tCO\tArchuleta County\tH1\n81029\t8009\tCampo\tCO\tBaca County\tH1\n81084\t8009\tTwo buttes\tCO\tBaca County\tH1\n81073\t8009\tSpringfield\tCO\tBaca County\tH1\n81090\t8009\tWalsh\tCO\tBaca County\tH1\n81047\t8009\tHolly\tCO\tBaca County\tH1\n81054\t8009\tLas animas\tCO\tBaca County\tH1\n81064\t8009\tPritchett\tCO\tBaca County\tH1\n81041\t8009\tGranada\tCO\tBaca County\tH1\n81087\t8009\tVilas\tCO\tBaca County\tH1\n81057\t8011\tMc clave\tCO\tBent County\tH1\n81044\t8011\tHasty\tCO\tBent County\tH1\n81050\t8011\tLa junta\tCO\tBent County\tH1\n81092\t8011\tWiley\tCO\tBent County\tH1\n81054\t8011\tLas animas\tCO\tBent County\tH1\n80533\t8013\tHygiene\tCO\tBoulder County\tH1\n80301\t8013\tBoulder\tCO\tBoulder County\tH1\n80544\t8013\tNiwot\tCO\tBoulder County\tH1\n80303\t8013\tBoulder\tCO\tBoulder County\tH1\n80513\t8013\tBerthoud\tCO\tBoulder County\tH1\n80422\t8013\tBlack hawk\tCO\tBoulder County\tH1\n80308\t8013\tBoulder\tCO\tBoulder County\tH1\n80502\t8013\tLongmont\tCO\tBoulder County\tH1\n80310\t8013\tBoulder\tCO\tBoulder County\tH1\n80305\t8013\tBoulder\tCO\tBoulder County\tH1\n80516\t8013\tErie\tCO\tBoulder County\tH1\n80466\t8013\tNederland\tCO\tBoulder County\tH1\n80510\t8013\tAllenspark\tCO\tBoulder County\tH1\n80309\t8013\tBoulder\tCO\tBoulder County\tH1\n80020\t8013\tBroomfield\tCO\tBoulder County\tH1\n80304\t8013\tBoulder\tCO\tBoulder County\tH1\n80503\t8013\tLongmont\tCO\tBoulder County\tH1\n80306\t8013\tBoulder\tCO\tBoulder County\tH1\n80021\t8013\tBroomfield\tCO\tBoulder County\tH1\n80027\t8013\tLouisville\tCO\tBoulder County\tH1\n80403\t8013\tGolden\tCO\tBoulder County\tH1\n80501\t8013\tLongmont\tCO\tBoulder County\tH1\n80481\t8013\tWard\tCO\tBoulder County\tH1\n80025\t8013\tEldorado springs\tCO\tBoulder County\tH1\n80026\t8013\tLafayette\tCO\tBoulder County\tH1\n80504\t8013\tLongmont\tCO\tBoulder County\tH1\n80302\t8013\tBoulder\tCO\tBoulder County\tH1\n80471\t8013\tPinecliffe\tCO\tBoulder County\tH1\n80455\t8013\tJamestown\tCO\tBoulder County\tH1\n80540\t8013\tLyons\tCO\tBoulder County\tH1\n80307\t8013\tBoulder\tCO\tBoulder County\tH1\n80314\t8013\tBoulder\tCO\tBoulder County\tH1\n80038\t8014\tBroomfield\tCO\tBroomfield County\tH6\n80516\t8014\tErie\tCO\tBroomfield County\tH6\n80020\t8014\tBroomfield\tCO\tBroomfield County\tH6\n80023\t8014\tBroomfield\tCO\tBroomfield County\tH6\n80234\t8014\tDenver\tCO\tBroomfield County\tH6\n80021\t8014\tBroomfield\tCO\tBroomfield County\tH6\n80027\t8014\tLouisville\tCO\tBroomfield County\tH6\n80603\t8014\tBrighton\tCO\tBroomfield County\tH6\n81236\t8015\tNathrop\tCO\tChaffee County\tH1\n81242\t8015\tPoncha springs\tCO\tChaffee County\tH1\n81201\t8015\tSalida\tCO\tChaffee County\tH1\n81251\t8015\tTwin lakes\tCO\tChaffee County\tH1\n81227\t8015\tMonarch\tCO\tChaffee County\tH1\n81211\t8015\tBuena vista\tCO\tChaffee County\tH1\n81228\t8015\tGranite\tCO\tChaffee County\tH1\n80825\t8017\tKit carson\tCO\tCheyenne County\tH1\n81045\t8017\tHaswell\tCO\tCheyenne County\tH1\n80810\t8017\tCheyenne wells\tCO\tCheyenne County\tH1\n81036\t8017\tEads\tCO\tCheyenne County\tH1\n80862\t8017\tWild horse\tCO\tCheyenne County\tH1\n80802\t8017\tArapahoe\tCO\tCheyenne County\tH1\n80439\t8019\tEvergreen\tCO\tClear Creek County\tH1\n80438\t8019\tEmpire\tCO\tClear Creek County\tH1\n80452\t8019\tIdaho springs\tCO\tClear Creek County\tH1\n80436\t8019\tDumont\tCO\tClear Creek County\tH1\n80476\t8019\tSilver plume\tCO\tClear Creek County\tH1\n80444\t8019\tGeorgetown\tCO\tClear Creek County\tH1\n81120\t8021\tAntonito\tCO\tConejos County\tH1\n81151\t8021\tSanford\tCO\tConejos County\tH1\n81101\t8021\tAlamosa\tCO\tConejos County\tH1\n81141\t8021\tManassa\tCO\tConejos County\tH1\n81140\t8021\tLa jara\tCO\tConejos County\tH1\n81124\t8021\tCapulin\tCO\tConejos County\tH1\n81129\t8021\tConejos\tCO\tConejos County\tH1\n81148\t8021\tRomeo\tCO\tConejos 
